vi "Add.vi"(8 "error in (no error)":errorcluster caption="错误输入（无错误）", 9 "Value":string, 10 "Key":string, 11 "Dictionary In":refnum<class "Dictionary.lvclass"> caption="DNL_LabVIEW Object in") -> (0 "error out":errorcluster caption="错误输出", 1 "Key Exist?":bool, 3 "Dictionary Out":refnum<class "Dictionary.lvclass"> caption="DNL_LabVIEW Object out")   [LabVIEW 2012, in "Dictionary.lvclass"]
uses:
  Dictionary.lvclass
  Dictionary.lvclass/Dictionary.ctl
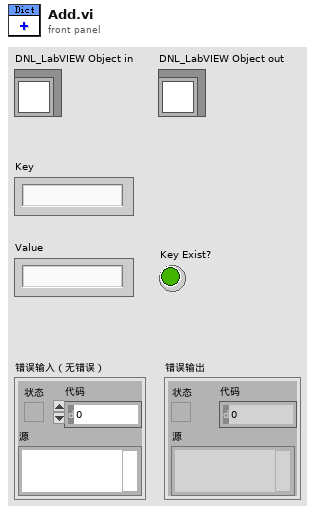
[diagram p1: front panel]
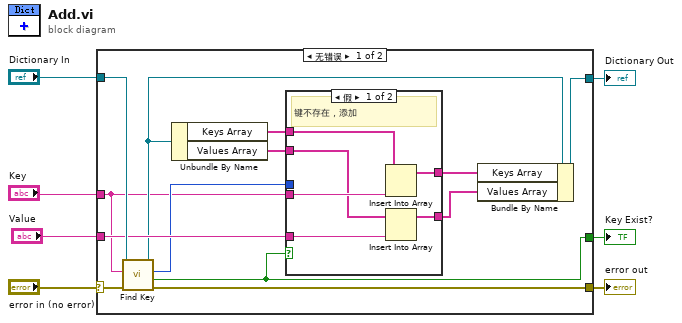
[diagram p0: block diagram]
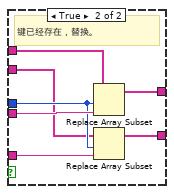
[diagram p2: hidden frame]
diagram:
  n1 = case shown="无错误" "error in (no error)" {
    selector: "error in (no error)" -> [w19 w35]
    tunnel: [w12 w35] -> w6
    tunnel: [w13 w34] -> w4
    tunnel: "Dictionary In" -> [w20 w34]
    tunnel: "Value" -> [w18 _]
    tunnel: "Key" -> [w10 _]
    tunnel: [w11 _] -> w1
    frame No Error {
      n2 = call "Find Key.vi"("error in (no error)"=w19, "Key"=w10, "Dictionary In"=w20) -> ("error out"=w12:errorcluster, "Key Exist?"=w11:bool, "Index"=w17:i32, "Dictionary Out"=w16:refnum<class "Dictionary.lvclass">)  [unwired: 5 in]
      n3 = Unbundle By Name(w16) -> ("Keys Array"=w9:string[], "Values Array"=w8:string[])
      n4 = case shown="假" w11 {
        tunnel: w18 -> [w23 w32]
        tunnel: w10 -> [w26 w33]
        tunnel: [w25 w29] -> w15
        tunnel: [w24 w30] -> w14
        tunnel: w17 -> [_ w31]
        tunnel: w9 -> [w22 w28]
        tunnel: w8 -> [w21 w27]
        frame False {
          # "键不存在，添加"
          n5 = Insert Into Array(array=w22, new element=w26) -> (w25:string[])  [unwired: 1 in]
          n6 = Insert Into Array(array=w21, new element=w23) -> (w24:string[])  [unwired: 1 in]
        }
        frame True {
          # "键已经存在，替换。"
          n7 = Replace Array Subset(array=w28, new element=w33, index=w31) -> (w29:string[])
          n8 = Replace Array Subset(array=w27, new element=w32, index=w31) -> (w30:string[])
        }
      }
      n9 = Bundle By Name(cluster=w16, "Keys Array"=w15, "Values Array"=w14) -> (w13:refnum<class "Dictionary.lvclass">)
    }
    frame Error {
    }
  }
  "error out" <- w6
  "Dictionary Out" <- w4
  "Key Exist?" <- w1
